vi "WS1050 Cycle Index Cmd.vi"(7 "Select Cycles Seq":u16(ring) items=["L_MSB", "M_LSB", "L_M_LSB", "M_L_MSB"], 8 "error in (no error)":errorcluster, 9 "Index":i32, 10 "OFF":string="00", 11 "ON":string[](array[string])=["38", "34", "30", "2C", "28", "24", "20", "1C", "18", "14", "10", "0C", "08", "04"]) -> (0 "error out":errorcluster, 1 "CMD OFF":string[](array[string]), 2 "CMD ON":string[](array[string]), 3 "Cmd To Cycles":string[](array[string]), 5 "Stress Beams":string)   [LabVIEW 2012]
panel:
  in  "Drivers":string[](array[string])=["B14", "B13", "B12", "B11", "B10", "B9", "B8", "B7", "B6", "B5", "B4", "B3", "B2", "B1"]
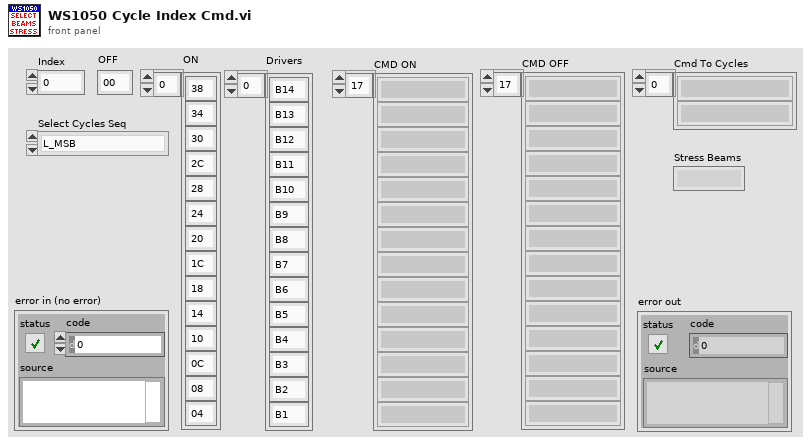
[diagram p1: front panel]
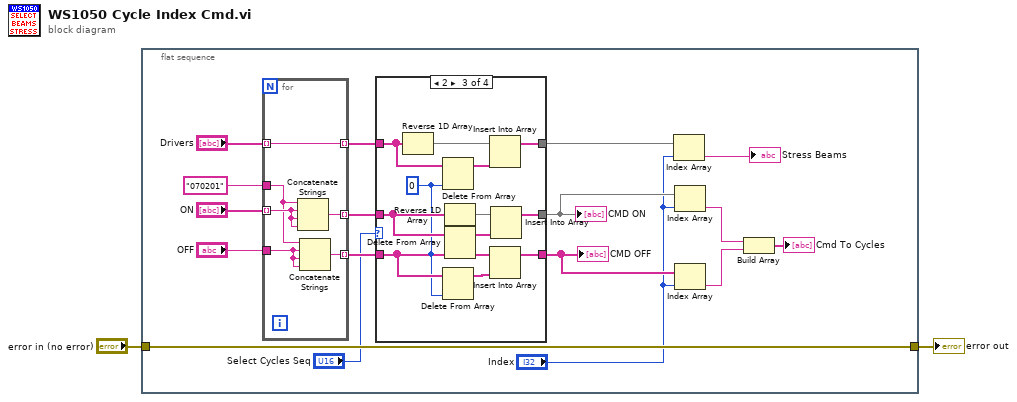
[diagram p0: block diagram]
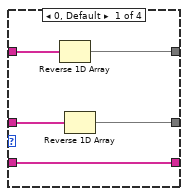
[diagram p2: hidden frame]
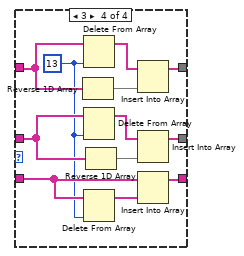
[diagram p4: hidden frame]
diagram:
  n1 = flat-sequence {
    tunnel: "error in (no error)" -> [w9]
    tunnel: [w9] -> w1
    frame #0 {
      n2 = for {
        tunnel: "ON" -> [w57] mode=indexing
        tunnel: "OFF" -> [w56]
        tunnel: "070201" ("string") -> [w55]
        tunnel: [w54] -> w16 mode=indexing
        tunnel: [w53] -> w15 mode=indexing
        tunnel: "Drivers" -> [w52] mode=indexing
        tunnel: [w52] -> w6 mode=indexing
        n3 = Concatenate Strings(w55, w57, w57, w57) -> (w54:string)
        n4 = Concatenate Strings(w55, w56, w56, w56) -> (w53:string)
      }
      n5 = case shown="2" "Select Cycles Seq" {
        tunnel: w16 -> [w24 w27 w32 w43]
        tunnel: w15 -> [w22 w26 w30 w42]
        tunnel: [w23 w27 w38 w49] -> w11
        tunnel: [w22 w26 w37 w51] -> w10
        tunnel: w6 -> [w21 w25 w34 w46]
        tunnel: [w20 w25 w36 w47] -> w5
        frame 0, Default {
          n6 = Reverse 1D Array(array=w21) -> (reversed array=w20:string[])
          n7 = Reverse 1D Array(array=w24) -> (reversed array=w23:string[])
        }
        frame 1 {
        }
        frame 2 {
          w28 = 0 ("index")
          n8 = Reverse 1D Array(array=w34) -> (reversed array=w35:string[])
          n9 = Delete From Array(array=w34, index=w28) -> (array with subset deleted=w33:string[])  [unwired: 1 in, 1 out]
          n10 = Delete From Array(array=w30, index=w28) -> (array with subset deleted=w29:string[])  [unwired: 1 in, 1 out]
          n11 = Reverse 1D Array(array=w32) -> (reversed array=w39:string[])
          n12 = Delete From Array(array=w32, index=w28) -> (array with subset deleted=w31:string[])  [unwired: 1 in, 1 out]
          n13 = Insert Into Array(array=w35, new element=w33) -> (w36:string[])  [unwired: 1 in]
          n14 = Insert Into Array(array=w30, new element=w29) -> (w37:string[])  [unwired: 1 in]
          n15 = Insert Into Array(array=w39, new element=w31) -> (w38:string[])  [unwired: 1 in]
        }
        frame 3 {
          w40 = 13 ("index")
          n16 = Reverse 1D Array(array=w46) -> (reversed array=w48:string[])
          n17 = Delete From Array(array=w46, index=w40) -> (array with subset deleted=w45:string[])  [unwired: 1 in, 1 out]
          n18 = Delete From Array(array=w43, index=w40) -> (array with subset deleted=w44:string[])  [unwired: 1 in, 1 out]
          n19 = Delete From Array(array=w42, index=w40) -> (array with subset deleted=w41:string[])  [unwired: 1 in, 1 out]
          n20 = Reverse 1D Array(array=w43) -> (reversed array=w50:string[])
          n21 = Insert Into Array(array=w45, new element=w48) -> (w47:string[])  [unwired: 1 in]
          n22 = Insert Into Array(array=w44, new element=w50) -> (w49:string[])  [unwired: 1 in]
          n23 = Insert Into Array(array=w42, new element=w41) -> (w51:string[])  [unwired: 1 in]
        }
      }
      "CMD OFF" <- w10
      "CMD ON" <- w11
      n24 = Index Array(array=w5, index="Index") -> (element=→"Stress Beams":string)
      n25 = Index Array(array=w11, index="Index") -> (element=w14:string)
      n26 = Index Array(array=w10, index="Index") -> (element=w13:string)
      n27 = Build Array(w14, w13) -> (→"Cmd To Cycles":string[])
    }
  }
  "error out" <- w1
